vi "Operator.vi"(11 "JoystickDevRef in 2":T1) -> ()   [LabVIEW 2016]
uses:
  <vilib>/Rock Robotics/WPI/Joystick/WPI_JoystickDevRef.ctl
  <vilib>/Rock Robotics/WPI/Joystick/WPI_JoystickDeviceEnum.ctl
  <vilib>/Rock Robotics/Network Tables/NT Write Numeric Array.vi
  <vilib>/Rock Robotics/Network Tables/NT Write Boolean Array.vi
  Robot Values.vi
  <vilib>/ptbypt/NI_PtbyPt.lvlib
panel:
  in  "Overdrive Power":dbl=1.0 format="%#_13g"
  out "JoystickDevRef out 2":T1
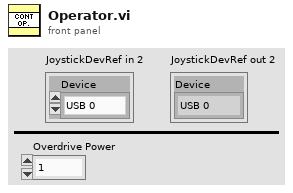
[diagram p1: front panel]
types:
  T1 = typedef "WPI_JoystickDevRef.ctl" = cluster{"Device":T2}
  T2 = typedef "WPI_JoystickDeviceEnum.ctl" = enum16{"USB 0", "USB 1", "USB 2", "USB 3", "USB 4", "USB 5"}
  T3 = typedef "Robot Values.ctl" = cluster{"Robot Drive":cluster{"Left Motor Power":dbl, "Right Motor Power":dbl, "Left Encoder Value":dbl, "Right Encoder Value":dbl, "High Gear?":bool, "PTO?":bool}, "Sensors":cluster{"Gyro Angle":u16, "Recalibrate Gyro":bool, "Reset Gyro":bool, "Ultrasonic":dbl}, "Shooter":cluster{"Prep Wheels":bool, "Shoot":bool, "Left Shooter Wheel Speed":dbl, "Wheels Moving":bool, "Shooter Prepped":bool, "Shooter RPS SP":dbl, "Shooting?":bool, "Left Shooter Wheel Power":dbl, "Right Shooter Wheel Power":dbl, "Acquisition Conveyor Power":dbl, "Hopper Beater Bar Power":dbl, "Filtered Left Shooter Speed":dbl, "Acquisition Motor Power":dbl, "Joystick Add":dbl, "D-Pad Add":dbl, "Shooter Use PID?":bool}, "Robot States":cluster{"Drive mode":string, "Alliance":T4, "Position":T5}, "Gear":cluster{"Ejection Active":bool}}
  T4 = typedef "WPI_DriverStationAllianceInfo.ctl" = enum16{"Red", "Blue", "Invalid"}
  T5 = typedef "WPI_DriverStationPositionInfo.ctl" = enum16{"1", "2", "3"}
  T6 = cluster{"Start  Button":bool, "Back Button":bool, "Left Trigger":bool, "Left  Bumper":bool, "Right Trigger":bool, "Right Bumper":bool, "A Button":bool, "B Button":bool, "X Button":bool, "Y Button":bool, "Left Joystick Press":bool, "Right Joystick Press":bool}
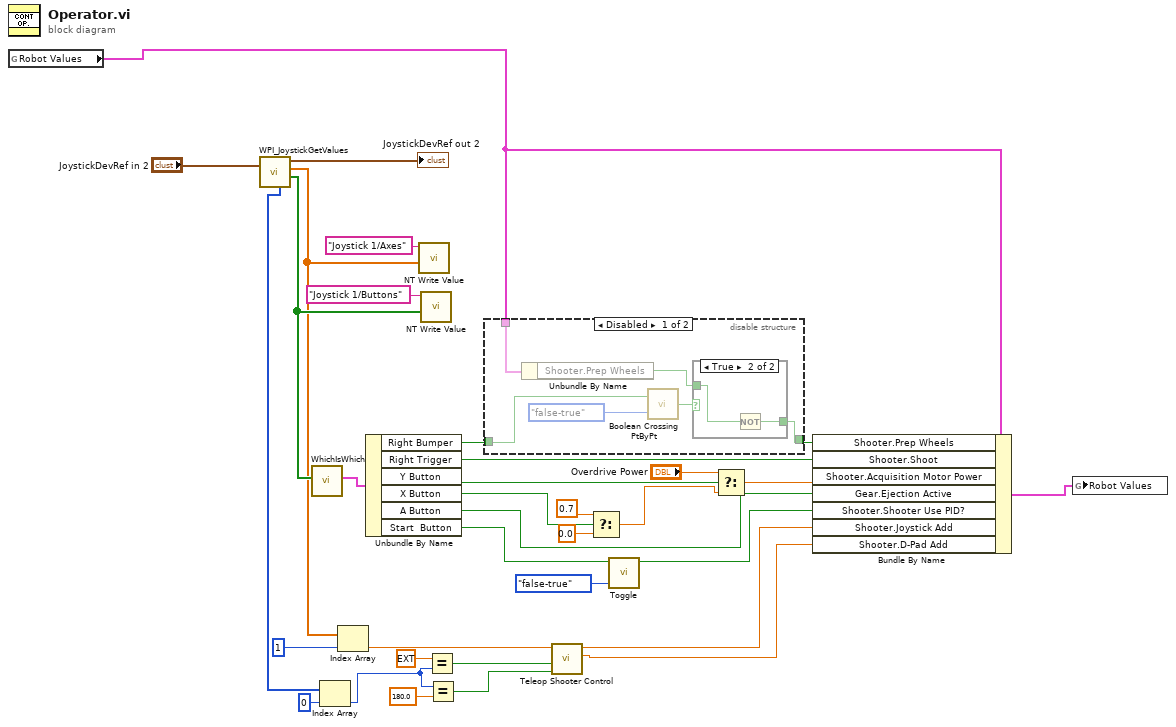
[diagram p0: block diagram]
diagram:
  n1 = global read "Robot Values.vi" "Robot Values"() -> (w12:T3)
  n2 = call <vilib>:"WPI_JoystickGetValues.vi"("JoystickDevRef"="JoystickDevRef in 2") -> ("Buttons"=w30:bool[], "Axes"=w16:dbl[], "JoystickDevRef"=→"JoystickDevRef out 2":T1, "POVs"=w4:i16[])  [unwired: 6 in, 1 out]
  n3 = call "WhichIsWhich.vi"("Button Values Array"=w30) -> ("Button Values Cluster"=w29:T6)  [unwired: 8 in]
  n4 = Index Array(array=w4, index=0) -> (element=w3:i16)
  n5 = Index Array(array=w16, index=1) -> (element=w14:dbl)
  n6 = Unbundle By Name(w29) -> ("Right Bumper"=w21:bool, "Right Trigger"=w28:bool, "Y Button"=w23:bool, "X Button"=w22:bool, "A Button"=w17:bool, "Start  Button"=w5:bool)
  n7 = call-poly <vilib>:"NT Write Value.vi"("Numeric Array"=w16, "Name"="Joystick 1/Axes") -> ()  [unwired: 9 in, 1 out]
  n8 = call-poly <vilib>:"NT Write Value.vi"("Boolean Array"=w30, "Name"="Joystick 1/Buttons") -> ()  [unwired: 9 in, 1 out]
  n9 = Equal?(x=ext 0.0, y=w3) -> (x = y?=w10:bool)
  n10 = Equal?(x=w3, y=180.0) -> (x = y?=w7:bool)
  n11 = disable-structure shown="Disabled" {
    disable-tunnel: w12 -> [w40 _]
    disable-tunnel: w21 -> [w39 w44]
    disable-tunnel: [w35 w44] -> w20
    frame Disabled {
      n12 = Unbundle By Name(w40) -> ("Shooter.Prep Wheels"=w36:bool)
      n13 = call <vilib>:"Boolean Crossing PtByPt.vi"("direction"=enum16{"either", "false-true", "true-false"}."false-true", "input"=w39) -> ("crossing"=w37:bool)  [unwired: 1 in]
      n14 = case shown="True" w37 {
        tunnel: w36 -> [w41 w43]
        tunnel: [w41 w42] -> w35
        frame False {
        }
        frame True {
          n15 = Not(x=w43) -> (.not. x?=w42:bool)
        }
      }
    }
    frame Enabled {
    }
  }
  n16 = call "Teleop Shooter Control.vi"("D-Pad Down Pressed?"=w7, "D-Pad Up Pressed?"=w10, "Joystick Value"=w14) -> ("D-Pad Output"=w11:dbl, "Joystick Output"=w13:dbl)  [unwired: 7 in]
  n17 = Select(t=0.7, s=w22, f=0.0) -> (s? t:f=w19:dbl)
  n18 = call "Toggle.vi"("direction"=enum16{"either", "false-true", "true-false"}."false-true", "Input"=w5) -> ("Output"=w1:bool)  [unwired: 9 in]
  n19 = Select(t="Overdrive Power", s=w23, f=w19) -> (s? t:f=w24:dbl)
  n20 = Bundle By Name(cluster=w12, "Shooter.Prep Wheels"=w20, "Shooter.Shoot"=w28, "Shooter.Acquisition Motor Power"=w24, "Gear.Ejection Active"=w17, "Shooter.Shooter Use PID?"=w1, "Shooter.Joystick Add"=w13, "Shooter.D-Pad Add"=w11) -> (w27:T3)
  n21 = global write "Robot Values.vi" "Robot Values"(w27) -> ()
